vi "Balancing.vi"() -> ()   [LabVIEW 2011]
uses:
  <vilib>/Rock Robotics/WPI/DriverStation/DriverStationLCD/WPI_DriverStationLCDLCDLine.ctl
  Robot Global Data.vi
  <vilib>/Analysis/NI_AALBase.lvlib
panel:
  out "ForAvg":dbl[](array[numeric])
  out "Balance Motor":dbl
  out "Current Angle Array":dbl[](array[numeric])
  out "Current Angle":dbl
  out "Balancing Gauge":dbl(knob) scale=-0.65..0.65
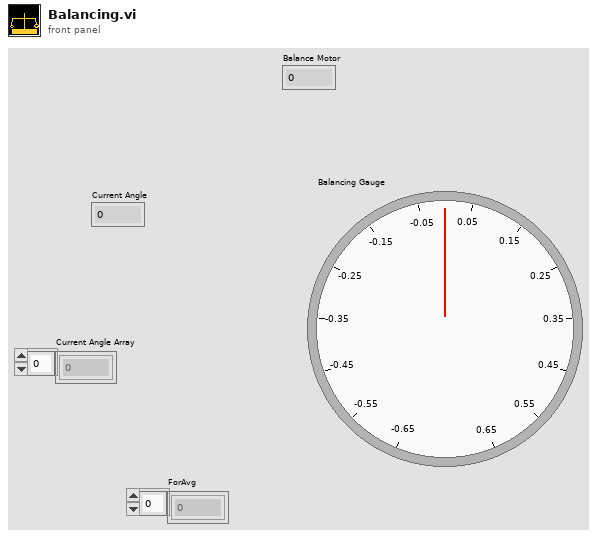
[diagram p1: front panel]
types:
  T1 = typedef "WPI_AnalogChannelDevRef.ctl" = cluster{"DevStatus":errorcluster, "Analog Module":T2, "Analog Channel":T3}
  T2 = typedef "FPGA_TypedefAnalogModule.ctl" = enum16{"Analog Module 1", "Analog Module 2"}
  T3 = typedef "FPGA_AIChannel.ctl" = enum8{"AI 1", "AI 2", "AI 3", "AI 4", "AI 5", "AI 6", "AI 7", "AI 8", "Invalid"}
  T4 = typedef "WPI_DriverStationLCDLCDLine.ctl" = enum16{"Main - Line 1", "User - Line 2", "User - Line 3", "User - Line 4", "User - Line 5", "User - Line 6"}
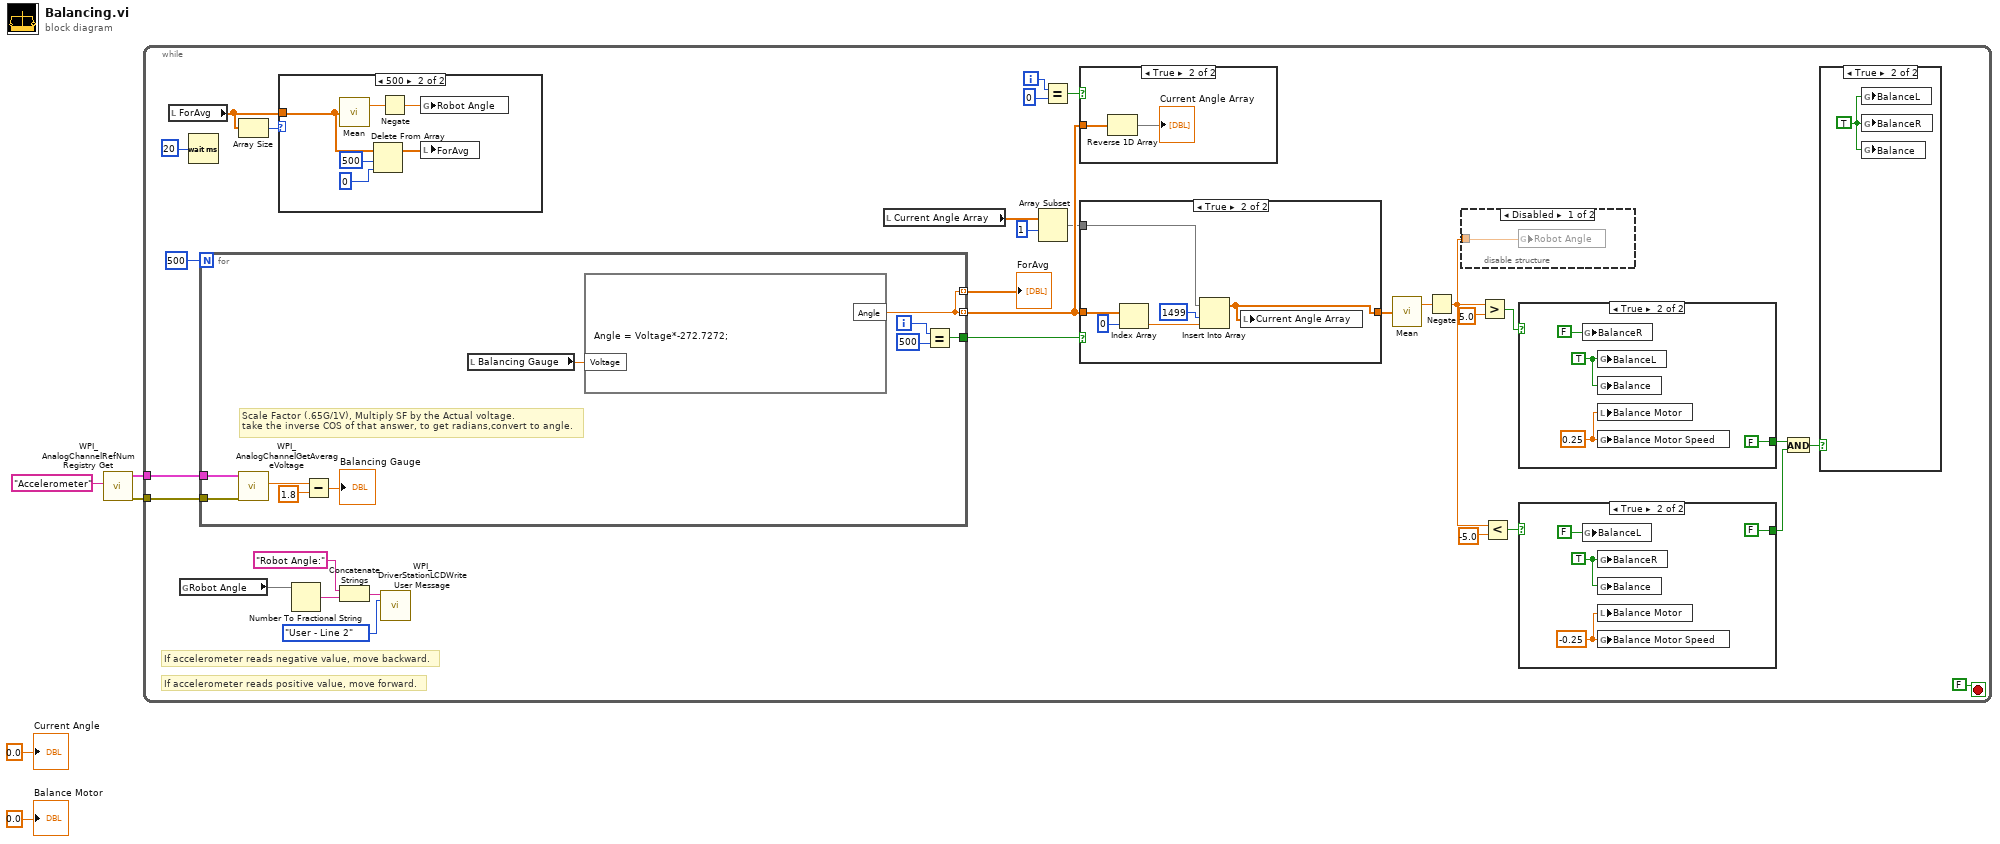
[diagram p0: block diagram]
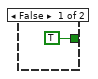
[diagram p7: hidden frame]
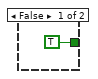
[diagram p8: hidden frame]
diagram:
  n1 = call <vilib>:"WPI_AnalogChannelRefNum Registry Get.vi"("refnum name"="Accelerometer") -> ("error out"=w1:errorcluster, "AIDeviceRef"=w2:T1)  [unwired: 9 in]
  n2 = while {
    tunnel: w2 -> [w12]
    tunnel: w1 -> [w11]
    i -> [w16]
    stop <- FALSE stop-if-true
    # "If accelerometer reads negative value, move backward."
    # "If accelerometer reads positive value, move forward."
    n3 = local read "ForAvg"() -> (w8:dbl[])
    n4 = global read "Robot Global Data.vi" "Robot Angle"() -> (w7)
    n5 = Wait (ms)(milliseconds to wait=u32 20) -> ()  [unwired: 1 out]
    n6 = for {
      N: 500 -> [_]
      tunnel: [w53] -> w22 mode=indexing
      tunnel: [w60] -> w23
      tunnel: w12 -> [w55]
      tunnel: w11 -> [w54]
      tunnel: [w53] -> w10 mode=indexing
      i -> [w59]
      # "Scale Factor (.65G/1V), Multiply SF by the Actual voltage.\ntake the inverse COS of that answer, to get radians,convert to angle."
      n7 = call <vilib>:"WPI_AnalogChannelGetAverageVoltage.vi"("error in (no error)"=w54, "AIDeviceRef"=w55) -> ("Voltage"=w58:dbl)  [unwired: 7 in, 2 out]
      n8 = Subtract(x=w58, y=1.8) -> (x-y=→"Balancing Gauge":dbl)
      n9 = local read "Balancing Gauge"() -> (w62:dbl)
      n10 = formula code="Angle = Voltage*-272.7272;"("Voltage"=w62) -> ("Angle"=w53:dbl)
      n11 = Equal?(x=w59, y=500) -> (x = y?=w60:bool)
    }
    "ForAvg" <- w10
    n12 = Array Size(array=w8) -> (size(s)=w9:i32)
    n13 = case shown="500" w9 {
      tunnel: w8 -> [_ w43]
      frame 0, Default {
      }
      frame 500 {
        n14 = call <vilib>:"Mean.vi"("X"=w43) -> ("mean"=w39:dbl)  [unwired: 1 out]
        n15 = Delete From Array(array=w43, length=500, index=0) -> (array with subset deleted=w42:dbl[])  [unwired: 1 out]
        n16 = Negate(x=w39) -> (-x=w38:dbl)
        n17 = global write "Robot Global Data.vi" "Robot Angle"(w38) -> ()
        n18 = local write "ForAvg"(w42) -> ()
      }
    }
    n19 = Number To Fractional String(number=w7) -> (F-format string=w30:string)  [unwired: 3 in]
    n20 = Concatenate Strings("Robot Angle:" ("string"), w30) -> (w29:string)
    n21 = call <vilib>:"WPI_DriverStationLCDWrite User Message.vi"("line text"=w29, "line"=WPI_DriverStationLCDLCDLine."User - Line 2") -> ()  [unwired: 13 in, 1 out]
    n22 = local read "Current Angle Array"() -> (w18:dbl[])
    n23 = Array Subset(array=w18, index=1) -> (w20:dbl[])  [unwired: 1 in]
    n24 = Equal?(x=w16, y=0) -> (x = y?=w14:bool)
    n25 = case shown="True" w14 {
      tunnel: w22 -> [_ w44]
      frame False {
      }
      frame True {
        n26 = Reverse 1D Array(array=w44) -> (reversed array=→"Current Angle Array":dbl[])
      }
    }
    n27 = case shown="True" w23 {
      tunnel: w20 -> [_ w51]
      tunnel: w22 -> [w46 w49]
      tunnel: [w46 w50] -> w21
      frame False {
      }
      frame True {
        n28 = Index Array(array=w49, index=0) -> (element=w47:dbl)
        n29 = Insert Into Array(array=w51, index=1499, new element=w47) -> (w50:dbl[])
        n30 = local write "Current Angle Array"(w50) -> ()
      }
    }
    n31 = call <vilib>:"Mean.vi"("X"=w21) -> ("mean"=w6:dbl)  [unwired: 1 out]
    n32 = Negate(x=w6) -> (-x=w13:dbl)
    n33 = disable-structure shown="Disabled" {
      disable-tunnel: w13 -> [w37 _]
      frame Disabled {
        n34 = global write "Robot Global Data.vi" "Robot Angle"(w37) -> ()
      }
      frame Enabled {
      }
    }
    n35 = Greater?(x=w13, y=5.0) -> (0:w34:bool)
    n36 = Less?(x=w13, y=-5.0) -> (x < y?=w33:bool)
    n37 = case shown="True" w34 {
      tunnel: [TRUE FALSE] -> w27
      frame False {
      }
      frame True {
        w70 = 0.25 ("Balance Motor")
        w73 = TRUE ("Balance")
        n38 = global write "Robot Global Data.vi" "BalanceR"(FALSE ("BalanceR")) -> ()
        n39 = global write "Robot Global Data.vi" "BalanceL"(w73) -> ()
        n40 = global write "Robot Global Data.vi" "Balance"(w73) -> ()
        n41 = local write "Balance Motor"(w70) -> ()
        n42 = global write "Robot Global Data.vi" "Balance Motor Speed"(w70) -> ()
      }
    }
    n43 = case shown="True" w33 {
      tunnel: [TRUE FALSE] -> w26
      frame False {
      }
      frame True {
        w65 = -0.25 ("Balance Motor")
        w68 = TRUE ("Balance")
        n44 = global write "Robot Global Data.vi" "BalanceL"(FALSE ("BalanceR")) -> ()
        n45 = global write "Robot Global Data.vi" "BalanceR"(w68) -> ()
        n46 = global write "Robot Global Data.vi" "Balance"(w68) -> ()
        n47 = local write "Balance Motor"(w65) -> ()
        n48 = global write "Robot Global Data.vi" "Balance Motor Speed"(w65) -> ()
      }
    }
    n49 = And(x=w27, y=w26) -> (x .and. y?=w28:bool)
    n50 = case shown="True" w28 {
      frame False {
      }
      frame True {
        w63 = TRUE ("Balance")
        n51 = global write "Robot Global Data.vi" "BalanceL"(w63) -> ()
        n52 = global write "Robot Global Data.vi" "BalanceR"(w63) -> ()
        n53 = global write "Robot Global Data.vi" "Balance"(w63) -> ()
      }
    }
  }
  "Current Angle" <- 0.0 ("Current Angle")
  "Balance Motor" <- 0.0 ("Balance Motor")
